vi "Serialize as XML.vi"(8 "error in (no error)":errorcluster, 11 "Attribute in":refnum<class "Attribute.lvclass">) -> (0 "error out":errorcluster, 2 "XML Fragment":string, 3 "Attribute out":refnum<class "Attribute.lvclass">)   [LabVIEW 2018, in "VILab.lvlib" / "Attribute.lvclass"]
uses:
  Attribute.lvclass
  Attribute.lvclass/Attribute.ctl
  Data Item.lvclass
  VILab.lvlib
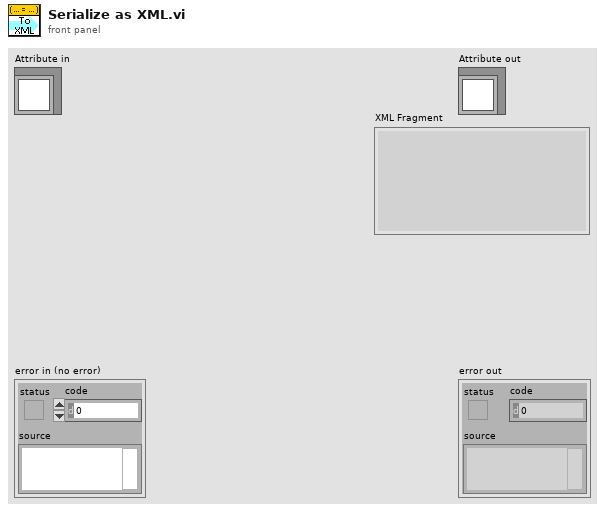
[diagram p1: front panel]
types:
  T1 = typedef "VILab.lvlib/Data Item.lvclass/Behavior Flags.ctl" = cluster{"Children":T2, "Editable":bool, "XML uses />":bool}
  T2 = typedef "VILab.lvlib/Data Item.lvclass/Child Support.ctl" = enum16{"None", "One", "At most one", "Multiple"}
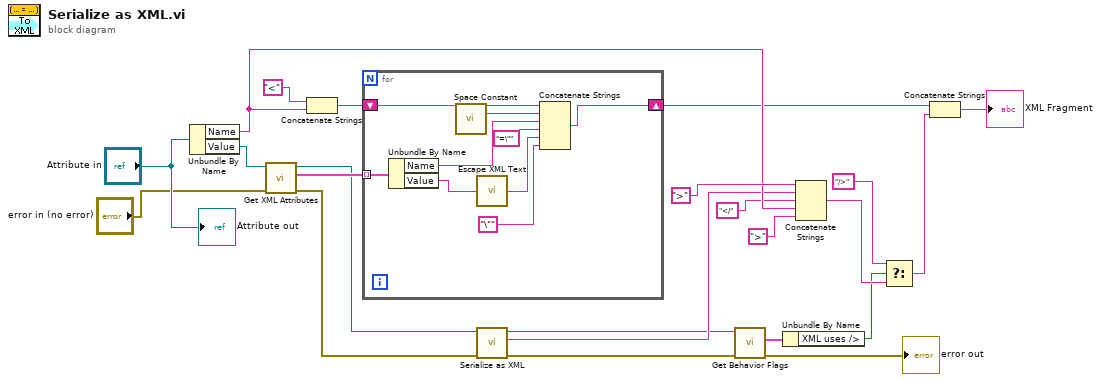
[diagram p0: block diagram]
diagram:
  n1 = Unbundle By Name("Attribute in") -> ("Name"=w18:string, "Value"=w14:refnum<class "Data Item.lvclass">)
  n2 = call-dynamic "Get XML Attributes.vi"("error in (no error)"="error in (no error)", "Data Item in"=w14) -> ("error out"=w19:errorcluster, "XML Attributes"=w21:cluster{"Name":string, "Value":string}[], "Data Item out"=w13:refnum<class "Data Item.lvclass">)  [unwired: 7 in]
  n3 = Concatenate Strings("<", w18) -> (w22:string)
  n4 = for {
    shift-right: [w30] -> w11
    shift-left: w22 -> [w31]
    tunnel: w21 -> [w32] mode=indexing
    n5 = Unbundle By Name(w32) -> ("Name"=w28:string, "Value"=w27:string)
    n6 = call <vilib>:"Space Constant.vi"() -> ("String"=w29:string)
    n7 = call "Escape XML Text.vi"("String"=w27) -> ("Escaped"=w25:string)
    n8 = Concatenate Strings(w31, w29, w28, "=\"", w25, "\"") -> (w30:string)
  }
  n9 = call-dynamic "Serialize as XML.vi"("error in (no error)"=w19, "Data Item in"=w13) -> ("error out"=w4:errorcluster, "XML Fragment"=w10:string, "Data Item out"=w5:refnum<class "Data Item.lvclass">)  [unwired: 7 in]
  n10 = call-dynamic "Get Behavior Flags.vi"("error in (no error)"=w4, "Data Item in"=w5) -> ("error out"=→"error out":errorcluster, "Behavior"=w2:T1)  [unwired: 7 in, 1 out]
  n11 = Unbundle By Name(w2) -> ("XML uses />"=w1:bool)
  n12 = Concatenate Strings(">", w10, "</", w18, ">") -> (w9:string)
  n13 = Select(t="/>", s=w1, f=w9) -> (s? t:f=w7:string)
  n14 = Concatenate Strings(w11, w7) -> (→"XML Fragment":string)
  "Attribute out" <- "Attribute in"
